vi "Format Key String Base.vi"(9 "Row Index":i32, 11 "Control Information Rows":string[][](array[string])) -> (3 "Key String":string)   [LabVIEW 2017, in "Localization.lvlib" / "Control Info.lvclass"]
doc: "Uses the current Control Information Row to create the string for the base Key String that will hold the value of the Alternate Text in the INI file.\n\nChoose Movement Consulting, LLC"
uses:
  Control Info.lvclass
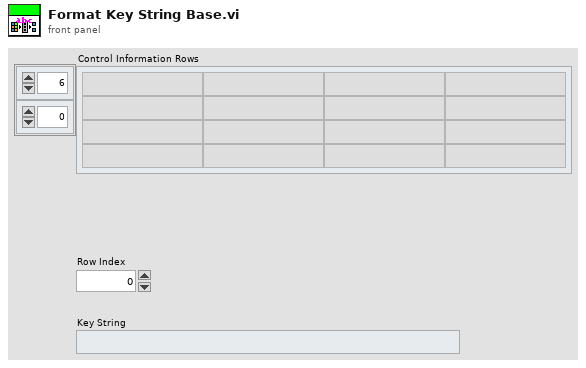
[diagram p1: front panel]
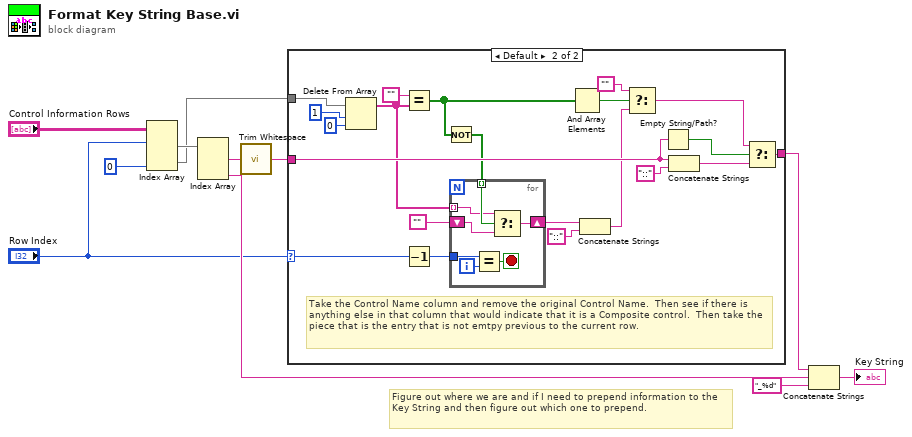
[diagram p0: block diagram]
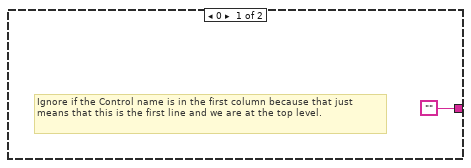
[diagram p2: hidden frame]
diagram:
  # "Figure out where we are and if I need to prepend information to the Key String and then figure out which one to prepend."
  n1 = Index Array(array="Control Information Rows", index (row) #1="Row Index", index (col) #2=0 ("index (row)")) -> (element #1=w4:string[], element #2=w1:string[])  [unwired: 2 in]
  n2 = Index Array(array=w4) -> (element #1=w9:string, element #3=w10:string)  [unwired: 3 in, 1 out]
  n3 = call <vilib>:"Trim Whitespace.vi"("string"=w9) -> ("trimmed string"=w6:string)  [unwired: 1 in]
  n4 = case shown="Default" "Row Index" {
    selector: "Row Index" -> [_ w19]
    tunnel: ["" w33] -> w11
    tunnel: w6 -> [_ w30]
    tunnel: w1 -> [_ w23]
    frame 0 {
      # "Ignore if the Control name is in the first column because that just means that this is the first line and we are at the top level."
    }
    frame Default {
      # "Take the Control Name column and remove the original Control Name.  Then see if there is anything else in that column that would indicate that it is a Composite control.  Then take the piece that is the entry that is not emtpy previous to the current row."
      n5 = Delete From Array(array=w23, length=1, index=0) -> (array with subset deleted=w20:string[])  [unwired: 1 out]
      n6 = Equal?(x="", y=w20) -> (x = y?=w17:bool[])
      n7 = Decrement(x=w19) -> (x-1=w18:i32)
      n8 = Not(x=w17) -> (.not. x?=w16:bool[])
      n9 = for {
        shift-right: [w38] -> w14
        shift-left: "" -> [w37]
        tunnel: w20 -> [w39] mode=indexing
        tunnel: w16 -> [w40] mode=indexing
        tunnel: w18 -> [w36]
        i -> [w35]
        stop <- w34 stop-if-true
        n10 = Equal?(x=w36, y=w35) -> (x = y?=w34:bool)
        n11 = Select(t=w39, s=w40, f=w37) -> (s? t:f=w38:string)
      }
      n12 = And Array Elements(Boolean array=w17) -> (logical AND=w25:bool)
      n13 = Concatenate Strings(w14, "::") -> (w13:string)
      n14 = Select(t="", s=w25, f=w13) -> (s? t:f=w22:string)
      n15 = Empty String/Path?(string/path=w30) -> (empty?=w29:bool)
      n16 = Concatenate Strings(w30, "::") -> (w32:string)
      n17 = Select(t=w22, s=w29, f=w32) -> (s? t:f=w33:string)
    }
  }
  n18 = Concatenate Strings(w11, w10, "_%d") -> (→"Key String":string)
